vi "Configure Voltage Output.vi"(0 "VISA resource name":refnum<visa-resource-name>, 1 "Voltage Bandwidth (0: High)":u16(ring) items=["High", "Low"], 5 "Voltage Immediate Amplitude (0 V)":dbl, 7 "Voltage Triggered Amplitude (0 V)":dbl, 9 "Voltage Slew (Inf)":dbl=inf, 11 "error in (no error)":errorcluster, 12 "Enable Current Priority (False)":bool, 13 "Current Priority Voltage Limit (25V)":dbl=25.0) -> (4 "VISA resource name out":refnum<visa-resource-name>, 15 "error out":errorcluster)   [LabVIEW 2019, in "Agilent N7976A.lvlib"]
doc: "Configures the output settings related to the voltage."
uses:
  <instrlib>/Agilent N7976A/Agilent N7976A.lvlib
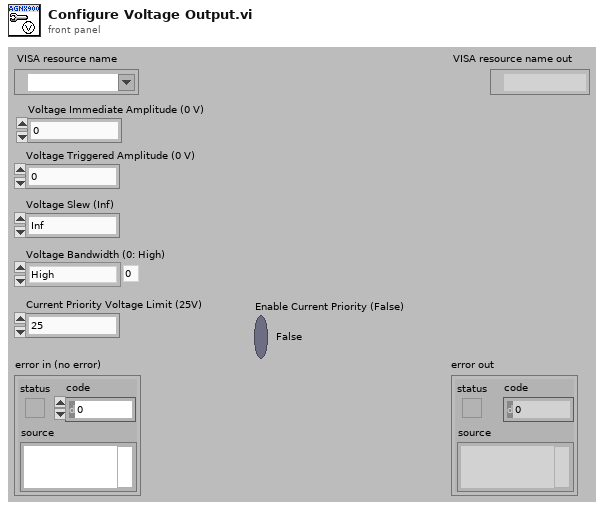
[diagram p1: front panel]
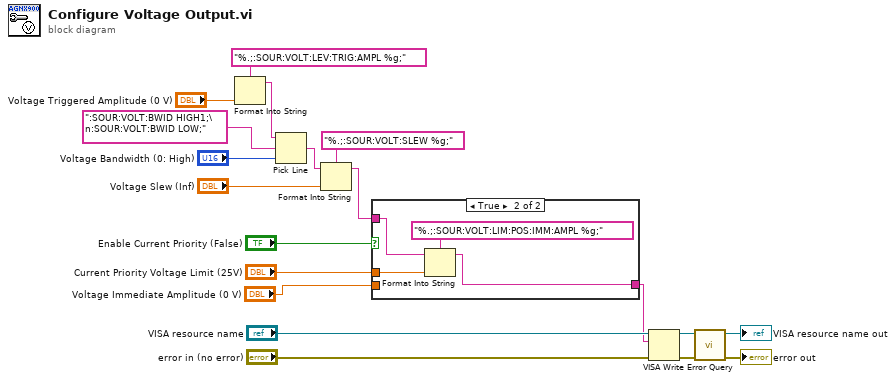
[diagram p0: block diagram]
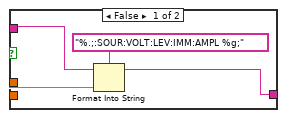
[diagram p2: hidden frame]
diagram:
  n1 = Format Into String(format string="%.;:SOUR:VOLT:LEV:TRIG:AMPL %g;", "Voltage Triggered Amplitude (0 V)") -> (resulting string=w2:string)  [unwired: 2 in, 1 out]
  n2 = Pick Line(string ("")=w2, multi-line string=":SOUR:VOLT:BWID HIGH1;\n:SOUR:VOLT:BWID LOW;", line index="Voltage Bandwidth (0: High)") -> (output string=w3:string)
  n3 = Format Into String(format string="%.;:SOUR:VOLT:SLEW %g;", initial string=w3, "Voltage Slew (Inf)") -> (resulting string=w4:string)  [unwired: 1 in, 1 out]
  n4 = case shown="True" "Enable Current Priority (False)" {
    tunnel: [w20 w27] -> w13
    tunnel: "Current Priority Voltage Limit (25V)" -> [_ w26]
    tunnel: w4 -> [w22 w24]
    tunnel: "Voltage Immediate Amplitude (0 V)" -> [w23 _]
    frame False {
      n5 = Format Into String(format string="%.;:SOUR:VOLT:LEV:IMM:AMPL %g;", initial string=w22, w23) -> (resulting string=w20:string)  [unwired: 1 in, 1 out]
    }
    frame True {
      n6 = Format Into String(format string="%.;:SOUR:VOLT:LIM:POS:IMM:AMPL %g;", initial string=w24, w26) -> (resulting string=w27:string)  [unwired: 1 in, 1 out]
    }
  }
  n7 = VISA Write(VISA resource name="VISA resource name", write buffer=w13, error in (no error)="error in (no error)") -> (VISA resource name out=w16:refnum<visa-resource-name>, error out=w17:errorcluster)  [unwired: 1 out]
  n8 = call <instrlib>:"Error Query.vi"("error in (no error)"=w17, "VISA resource name"=w16) -> ("error out"=→"error out":errorcluster, "VISA resource name out"=→"VISA resource name out":refnum<visa-resource-name>)  [unwired: 6 in, 2 out]
